vi "Add.vi"(1 "B":T1={"Array Num"=[1, 2, 3], "Decimal Index"=0, "stop"=FALSE}, 2 "A":T1={"Array Num"=[1, 2, 3], "Decimal Index"=0, "stop"=FALSE}) -> (0 "A+B":T1={"Array Num"=[1, 2, 3], "Decimal Index"=0, "stop"=FALSE})   [LabVIEW 2025]
uses:
  Number.ctl
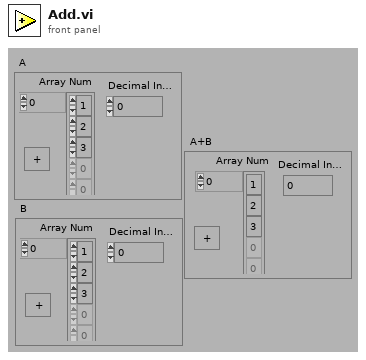
[diagram p1: front panel]
types:
  T1 = typedef "Number.ctl" = cluster{"Array Num":i8[], "Decimal Index":i32, "stop":bool}
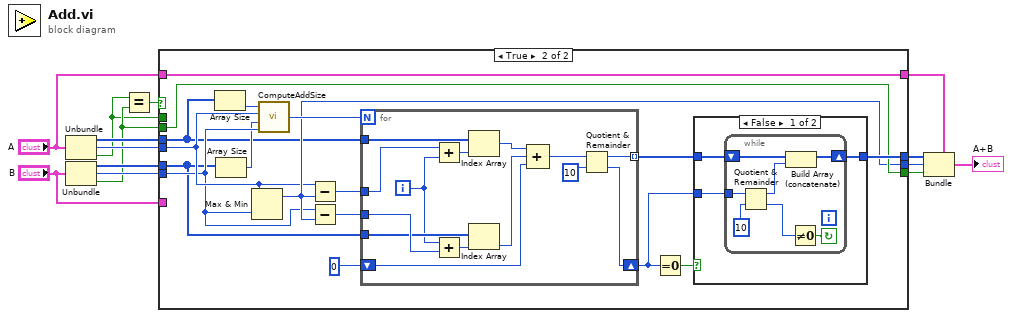
[diagram p0: block diagram]
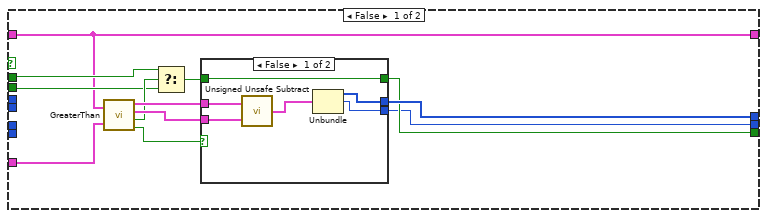
[diagram p2: hidden frame]
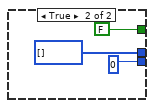
[diagram p3: hidden frame]
diagram:
  n1 = Unbundle("A") -> ("Array Num"=w12:i8[], "Decimal Index"=w13:i32, "stop"=w8:bool)
  n2 = Unbundle("B") -> ("Array Num"=w11:i8[], "Decimal Index"=w14:i32, "stop"=w9:bool)
  n3 = Equal?(x=w8, y=w9) -> (x = y?=w10:bool)
  n4 = case shown="True" w10 {
    tunnel: w11 -> [_ w39]
    tunnel: w12 -> [_ w36]
    tunnel: w13 -> [_ w42]
    tunnel: w14 -> [_ w41]
    tunnel: w9 -> [w22 w49]
    tunnel: w8 -> [w23 _]
    tunnel: [w19 w50] -> w7
    tunnel: [w17 w43] -> w6
    tunnel: [w18 w49] -> w5
    tunnel: "A" -> [w15 w40]
    tunnel: "B" -> [w16 _]
    tunnel: [w15 w40] -> w1
    frame False {
      n5 = call "GreaterThan.vi"("A"=w15, "B"=w16) -> ("Larger"=w26:T1, "Smaller"=w25:T1, "A Greater"=w24:bool, "Equal"=w21:bool)
      n6 = Select(t=w23, s=w24, f=w22) -> (s? t:f=w20:bool)
      n7 = case shown="False" w21 {
        tunnel: w25 -> [w27 _]
        tunnel: w26 -> [w28 _]
        tunnel: w20 -> [w32 _]
        tunnel: [w30 i8[] []] -> w19
        tunnel: [w29 0] -> w17
        tunnel: [w32 FALSE] -> w18
        frame False {
          n8 = call "Unsigned Unsafe Subtract.vi"("B"=w27, "A"=w28) -> ("A-B"=w31:T1)
          n9 = Unbundle(w31) -> ("Array Num"=w30:i8[], "Decimal Index"=w29:i32)  [unwired: 1 out]
        }
        frame True {
        }
      }
    }
    frame True {
      n10 = Array Size(array=w36) -> (size(s)=w37:i32)
      n11 = Array Size(array=w39) -> (size(s)=w38:i32)
      n12 = Max & Min(x=w42, y=w41) -> (max(x,y)=w43:i32)  [unwired: 1 out]
      n13 = call "ComputeAddSize.vi"("B Position"=w41, "B Array Size"=w38, "A Position"=w42, "A Array Size"=w37) -> ("Digits"=w47:i32)
      n14 = Subtract(x=w42, y=w43) -> (x-y=w46:i32)
      n15 = Subtract(x=w41, y=w43) -> (x-y=w45:i32)
      n16 = for {
        N: w47 -> [_]
        shift-right: [w54] -> w48
        shift-left: i8 0 -> [w66]
        tunnel: w46 -> [w57]
        tunnel: w45 -> [w62]
        tunnel: w39 -> [w60]
        tunnel: w36 -> [w59]
        tunnel: [w53] -> w44 mode=indexing
        i -> [w58]
        n17 = Add(x=w57, y=w58) -> (x+y=w61:i32)
        n18 = Add(x=w58, y=w62) -> (x+y=w63:i32)
        n19 = Index Array(array=w59, index=w61) -> (element=w64:i8)
        n20 = Index Array(array=w60, index=w63) -> (element=w65:i8)
        n21 = Compound Arithmetic op=ADD(w64, w65, w66) -> (w56:i8)
        n22 = Quotient & Remainder(x=w56, y=i8 10) -> (x-y*floor(x/y)=w53:i8, floor(x/y)=w54:i8)
      }
      n23 = Equal To 0?(x=w48) -> (x = 0?=w52:bool)
      n24 = case shown="False" w52 {
        tunnel: w44 -> [w69 w77]
        tunnel: [w68 w77] -> w50
        tunnel: w48 -> [w67 _]
        frame False {
          n25 = while {
            tunnel: w67 -> [w76]
            shift-right: [w72] -> w68
            shift-left: w69 -> [w71]
            stop <- w74 continue-if-true
            n26 = Quotient & Remainder(x=w76, y=i8 10) -> (x-y*floor(x/y)=w70:i8, floor(x/y)=w73:i8)
            n27 = Build Array (concatenate)(w71, w70) -> (w72:i8[])
            n28 = Not Equal To 0?(x=w73) -> (x != 0?=w74:bool)
          }
        }
        frame True {
        }
      }
    }
  }
  n29 = Bundle(cluster=w1, "Array Num"=w7, "Decimal Index"=w6, "stop"=w5) -> (→"A+B":T1)
